vi "python_control_power_write&read.vi"() -> ()   [LabVIEW 2024]
panel:
  out "返回值":T1
  in  "channel":dbl=1.0
  in  "current":dbl=1.0
  in  "voltage":dbl=3.0
  in  "visa_address":string="USB0::0xFFFF::0x6300::802071092796770281::INSTR"
  in  "函数名称":string
  in  "模块路径":path
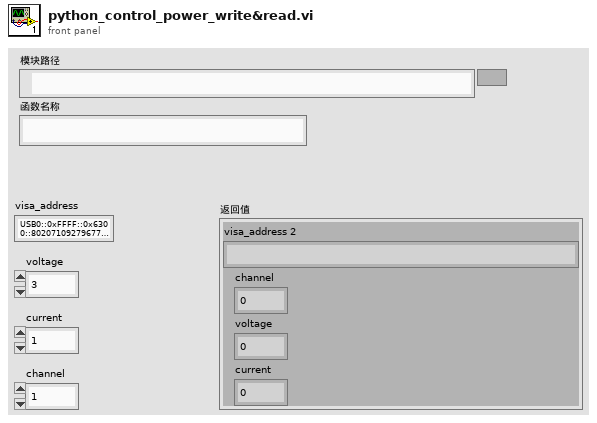
[diagram p1: front panel]
types:
  T1 = cluster{"visa_address 2":string, "channel":dbl, "voltage":dbl, "current":dbl}
  T2 = cluster{"visa_address 2":string, "current 2":dbl, "voltage 2":dbl, "channel 2":dbl}
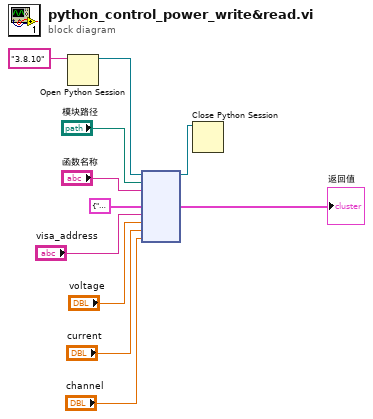
[diagram p0: block diagram]
diagram:
  n1 = Open Python Session(python version="3.8.10" ("Python版本")) -> (session out=w11:refnum<k35>)  [unwired: 2 in, 1 out]
  n2 = node(w11, "模块路径", "函数名称", T2 {"visa_address 2"="USB0::0xFFFF::0x6300::802071092796770281::INSTR", "current 2"=3.0, "voltage 2"=1.0, "channel 2"=1.0} ("簇"), "visa_address", "voltage", "current", "channel") -> (w10:refnum<k35>, →"返回值":T2)  [unwired: 5 in, 3 out]
  n3 = Close Python Session(session in=w10) -> ()  [unwired: 1 in, 1 out]
